vi "WPI_CounterDigitalInputToDigitalSource.vi"(3 "DigitalInputDevRef":T1={"DevStatus"={"status"=FALSE, "code"=0, "source"=""}, "DIO Channel"=enum."DIO 1"}) -> (7 "Digital Source":T3={"DevStatus"={"status"=FALSE, "code"=0, "source"=""}, "AnalogTriggerMode?"=FALSE, "DigitalMode"={"DIO Channel"=enum."DIO 1"}, "AnalogTriggerMode"={"AnalogTriggerIndex"=enum."Trig 0", "OutputType"=enum."InWindow"}})   [LabVIEW 2017]
doc: "Converts a digital input reference to a digital source reference. Wire the <B>Digital Source</B> output of this VI to VIs that require a digital source, such as the Open VIs on the Counter and Encoder palettes.\n\nThis software is licensed. Open the labview\\readme\\WPI Robotics Library Open Source License.txt file for more information."
uses:
  <vilib>/Rock Robotics/SystemInterfaces/CounterEncoderSourceConvertion/FPGA_CounterEncoderSourceConvertionLVSourceType.ctl
  <vilib>/Rock Robotics/SystemInterfaces/DIO/FPGA_DIODigitalSourceChannel.ctl
  <vilib>/Rock Robotics/SystemInterfaces/AnalogTrigger/FPGA_AnalogTriggerIndex.ctl
  <vilib>/Rock Robotics/SystemInterfaces/AnalogTrigger/FPGA_AnalogTriggerOutType.ctl
  <vilib>/Rock Robotics/WPI/DigitalInput/WPI_DigitalInputDevRef.ctl
  <vilib>/Rock Robotics/SystemInterfaces/DIO/FPGA_DIOChannel.ctl
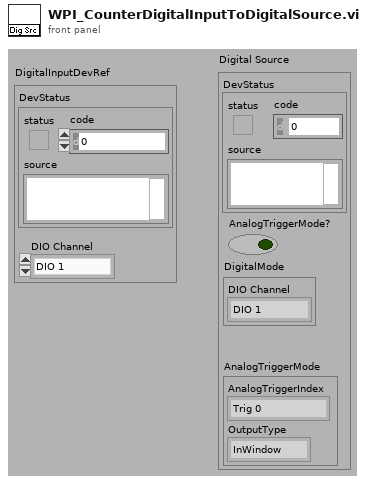
[diagram p1: front panel]
types:
  T1 = typedef "WPI_DigitalInputDevRef.ctl" = cluster{"DevStatus":errorcluster, "DIO Channel":T2}
  T2 = typedef "FPGA_DIOChannel.ctl" = enum8{"DIO 0", "DIO 1", "DIO 2", "DIO 3", "DIO 4", "DIO 5", "DIO 6", "DIO 7", "DIO 8", "DIO 9", "DIO MXP 0", "DIO MXP 1", "DIO MXP 2", "DIO MXP 3", "DIO MXP 4", "DIO MXP 5", "DIO MXP 6", "DIO MXP 7", "DIO MXP 8", "DIO MXP 9", "DIO MXP 10", "DIO MXP 11", "DIO MXP 12", "DIO MXP 13", "DIO MXP 14", "DIO MXP 15", "SPI Port CS1", "SPI Port CS2", "SPI Port CS3", "SPI Port MISO", "SPI Port MOSI", "Invalid"}
  T3 = typedef "FPGA_CounterEncoderSourceConvertionLVSourceType.ctl" = cluster{"DevStatus":errorcluster, "AnalogTriggerMode?":bool, "DigitalMode":cluster{"DIO Channel":T4}, "AnalogTriggerMode":cluster{"AnalogTriggerIndex":T5, "OutputType":T6}}
  T4 = typedef "FPGA_DIODigitalSourceChannel.ctl" = enum8{"DIO 0", "DIO 1", "DIO 2", "DIO 3", "DIO 4", "DIO 5", "DIO 6", "DIO 7", "DIO 8", "DIO 9", "DIO MXP 0", "DIO MXP 1", "DIO MXP 2", "DIO MXP 3", "DIO MXP 4", "DIO MXP 5", "DIO MXP 6", "DIO MXP 7", "DIO MXP 8", "DIO MXP 9", "DIO MXP 10", "DIO MXP 11", "DIO MXP 12", "DIO MXP 13", "DIO MXP 14", "DIO MXP 15", "SPI Port CS1", "SPI Port CS2", "SPI Port CS3", "SPI Port MISO", "SPI Port MOSI", "Disabled"}
  T5 = typedef "FPGA_AnalogTriggerIndex.ctl" = enum8{"Trig 0", "Trig 1", "Trig 2", "Trig 3", "Trig 4", "Trig 5", "Trig 6", "Trig 7", "Invalid"}
  T6 = typedef "FPGA_AnalogTriggerOutType.ctl" = enum16{"InWindow", "TriggerState", "Rising", "Falling"}
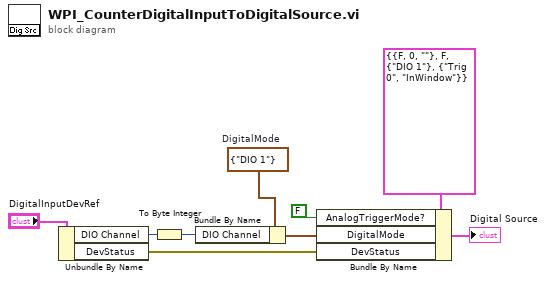
[diagram p0: block diagram]
diagram:
  w3 = cluster{"DIO Channel":T4} {"DIO Channel"=enum."DIO 1"}  # DigitalMode
  n1 = Unbundle By Name("DigitalInputDevRef") -> ("DIO Channel"=w6:T2, "DevStatus"=w1:errorcluster)
  n2 = To Byte Integer(number=w6) -> (8bit integer=w2:i8)
  n3 = Bundle By Name(cluster=w3, "DIO Channel"=w2) -> (w4:cluster{"DIO Channel":T4})
  n4 = Bundle By Name(cluster=T3 {"DevStatus"={"status"=FALSE, "code"=0, "source"=""}, "AnalogTriggerMode?"=FALSE, "DigitalMode"={"DIO Channel"=enum."DIO 1"}, "AnalogTriggerMode"={"AnalogTriggerIndex"=enum."Trig 0", "OutputType"=enum."InWindow"}} ("Up Source"), "AnalogTriggerMode?"=FALSE, "DigitalMode"=w4, "DevStatus"=w1) -> (→"Digital Source":T3)
